vi "Fetch Waveform With HZOffset.vi"(0 "VISA resource name":refnum<visa-resource-name>, 1 "First point (0: First point)":i32, 3 "Number of points (0: All points)":i32, 5 "Source (0: Channel 1)":u16(ring) items=["Channel 1", "Channel 2", "Channel 3", "Channel 4", "Memory 1", "Memory 2", "Memory 3", "Memory 4", "Function 1", "Function 2", "Function 3", "Function 4", "Function 5", "Function 6", "Function 7", "Function 8", "Other"], 9 "Timeout (10000 ms)":u32=10000, 10 "Custom Source ID":string, 11 "error in (no error)":errorcluster, 12 "Segment number (0: All segment)":i16, 14 "Sparsing (0: Every point)":i32) -> (4 "VISA resource name out":refnum<visa-resource-name>, 6 "Waveform Graph":waveform(dbl)(graph), 8 "error out":errorcluster, 15 "Horizontal Offset":dbl)   [LabVIEW 2022 SP3]
doc: "Returns the waveform the oscilloscope acquired for the specified channel. The waveform is from an acquisition that you initiate prior to calling this VI.\n\nYou use the Initiate VI to start an acquisition on the channels that you enable with the <B>Configure Channel</B> VI. The oscilloscope acquires waveforms for the enabled channels concurrently. You must call this VI separately for each enabled channel to obtain the waveforms.\n\nYou can call the <B>lcwave Read Single Waveform</B> VI or <B>lcwave Read Multiple Waveforms</B> VI instead of using low level VIs.\n\n<B>Note</B> This VI does not check the instrument status. Typically, you call this VI only in a sequence of calls to other low-level instrument driver VIs. The sequence performs one operation. You use the low-level VIs to optimize one or more aspects of interaction with the instrument."
uses:
  <instrlib>/LeCroy Wave Series/LeCroy Wave Series.lvlib
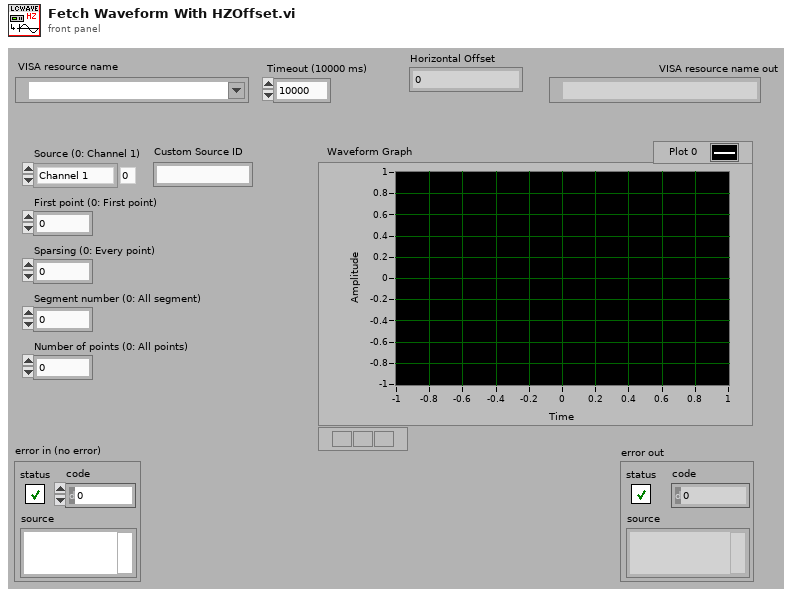
[diagram p1: front panel]
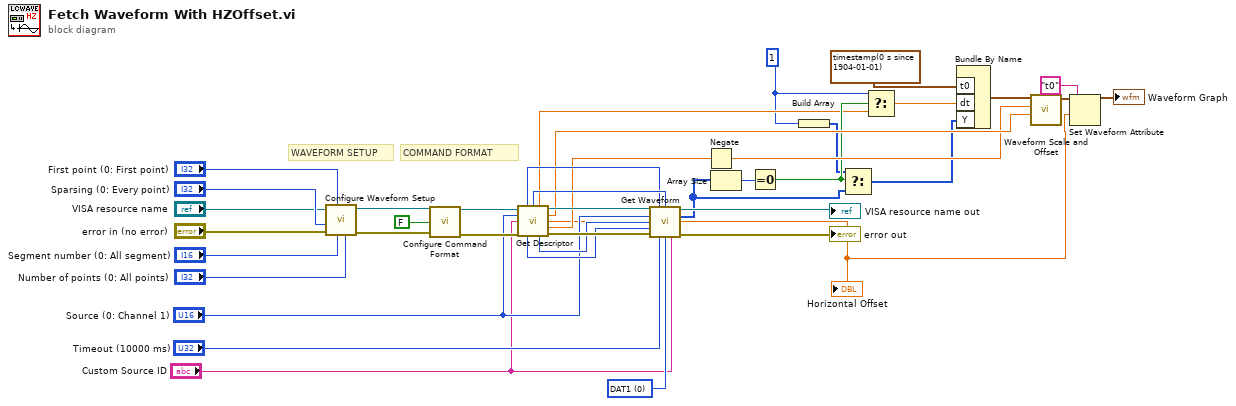
[diagram p0: block diagram]
diagram:
  w2 = i16 1
  w30 = u16 0 items=["DAT1", "DAT2"] ("Array (1: DAT1)")
  # "WAVEFORM SETUP"
  # "COMMAND FORMAT"
  n1 = call <instrlib>:"Configure Waveform Setup.vi"("Number of points (0: All points)"="Number of points (0: All points)", "Segment number (0: All segment)"="Segment number (0: All segment)", "First point (0: First point)"="First point (0: First point)", "error in (no error)"="error in (no error)", "Sparsing (0: Every point)"="Sparsing (0: Every point)", "VISA resource name"="VISA resource name") -> ("error out"=w34:errorcluster, "VISA resource name out"=w35:refnum<visa-resource-name>)  [unwired: 4 in]
  n2 = call <instrlib>:"Configure Command Format.vi"("VISA resource name"=w35, "Command format (T: Byte)"=FALSE, "error in (no error)"=w34) -> ("VISA resource name out"=w28:refnum<visa-resource-name>, "error out"=w27:errorcluster)  [unwired: 11 in]
  n3 = call <instrlib>:"Get Descriptor.vi"("VISA resource name"=w28, "Source (0: Channel 1)"="Source (0: Channel 1)", "Custom Source ID"="Custom Source ID", "error in (no error)"=w27) -> ("First Valid Point"=w24:i32, "Last Valid Point"=w25:i32, "Horizontal interval"=w3:sgl, "VISA resource name out"=w40:refnum<visa-resource-name>, "Vertical gain"=w21:sgl, "Horizontal Offset"=w9:dbl, "Vertical offset"=w20:sgl, "Number Of Data Points"=w29:i32, "Command type"=w36:i16, "error out"=w39:errorcluster)  [unwired: 1 in, 1 out]
  "Horizontal Offset" <- w9
  n4 = call <instrlib>:"Get Waveform.vi"("VISA resource name"=w40, "First Valid Point"=w24, "Last Valid Point"=w25, "Source (0: Channel 1)"="Source (0: Channel 1)", "Command type (0: byte)"=w36, "Number Of Data Points (10000)"=w29, "error in (no error)"=w39, "Timeout (10000 ms)"="Timeout (10000 ms)", "Array (0: DAT1)"=w30, "Custom Source ID"="Custom Source ID") -> ("VISA resource name out"=→"VISA resource name out":refnum<visa-resource-name>, "Waveform Graph"=w7:i16[], "error out"=→"error out":errorcluster)  [unwired: 3 in]
  n5 = Negate(x=w20) -> (-x=w19:sgl)
  n6 = Array Size(array=w7) -> (size(s)=w8:i32)
  n7 = Equal To 0?(x=w8) -> (x = 0?=w4:bool)
  n8 = Build Array(w2) -> (w1:i16[])
  n9 = Select(t=w1, s=w4, f=w7) -> (s? t:f=w6:i16[])
  n10 = Select(t=w2, s=w4, f=w3) -> (s? t:f=w5:sgl)
  n11 = Bundle By Name ("Build Waveform")("t0"=timestamp(0 s since 1904-01-01), "dt"=w5, "Y"=w6) -> (w23:waveform(i16))  [unwired: 1 in]
  n12 = call <vilib>:"Waveform Scale and Offset.vi"("scale"=w21, "offset"=w19, "waveform in"=w23) -> ("waveform out"=w22:waveform(dbl))  [unwired: 7 in, 1 out]
  n13 = Set Waveform Attribute(5:w9, 6:"t0" ("name"), 7:w22) -> (3:→"Waveform Graph":waveform(dbl))  [unwired: 1 in, 2 out]
